vi "ClassPanel.vi"(8 "error in (no error)":errorcluster caption="entrée d'erreur (pas d'erreur)", 11 "ESP301.lvclass":refnum<class "ESP301.lvclass">) -> (0 "error out":errorcluster caption="sortie d'erreur", 3 "ESP301.lvclass Out":refnum<class "ESP301.lvclass">)   [LabVIEW 2019, in "ESP301.lvclass"]
uses:
  ESP301.lvclass
  C:/Programmes Labview/LabScanV1A/DevicesClass/BaseDevice/BaseDevice.lvclass
  ESP301.lvclass/ESP301.ctl
  BaseDevice/ClassQueueMess.ctl
  BaseDevice/Accessor/GetClassEvent.vi
panel:
  out "APDs":bool
  in  "Con/Disc.":bool
  in  "Enable":bool
  in  "Home":bool caption="MiseAJour"
  out "Moving":bool
  out "Axis Model":string
  out "Valid Ref":bool
  out "BKD Lim":bool
  out "FWD Lim":bool
  in  "Axis":u8(ring)=1 items=["1"=1, "2"=2, "3"=3]
  out "ActPos":dbl=60.0 caption="Actual Pos(mm)" min=0.1 step=0.1 format="%#.4f"
  in  "Target":dbl caption="Target(mm)" min=-25000.0 max=25000.0 step=0.0001 format="%#.4f"
  in  "Axis Name":string
  in  "MainProgQ":refnum<queue>
  in  "MainProgQEvent":refnum<user-event>
  in  "Acq":bool
  in  "Stop":bool
  in  "StopMotion":bool caption="MiseAJour"
  out "Init Program":bool
  # "this MUST labeled with class name"
  # "this MUST be present and labeled \"Stop\" and \"Acq\""
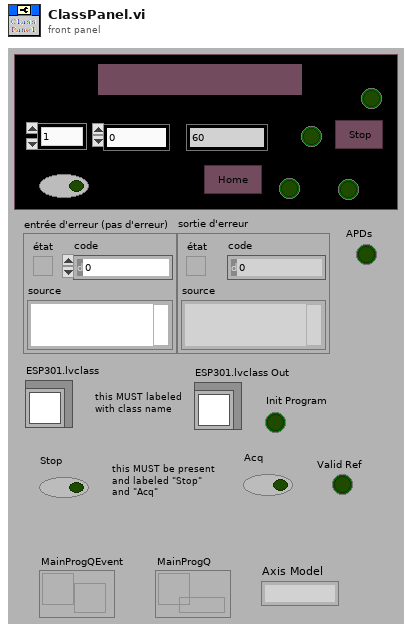
[diagram p1: front panel]
types:
  T1 = cluster{"ESP300mm":refnum<vi>, "ESP300ps":refnum<vi>, "MvgESP300":refnum<vi>}
  T2 = typedef "ClassQueueMess.ctl" = u16
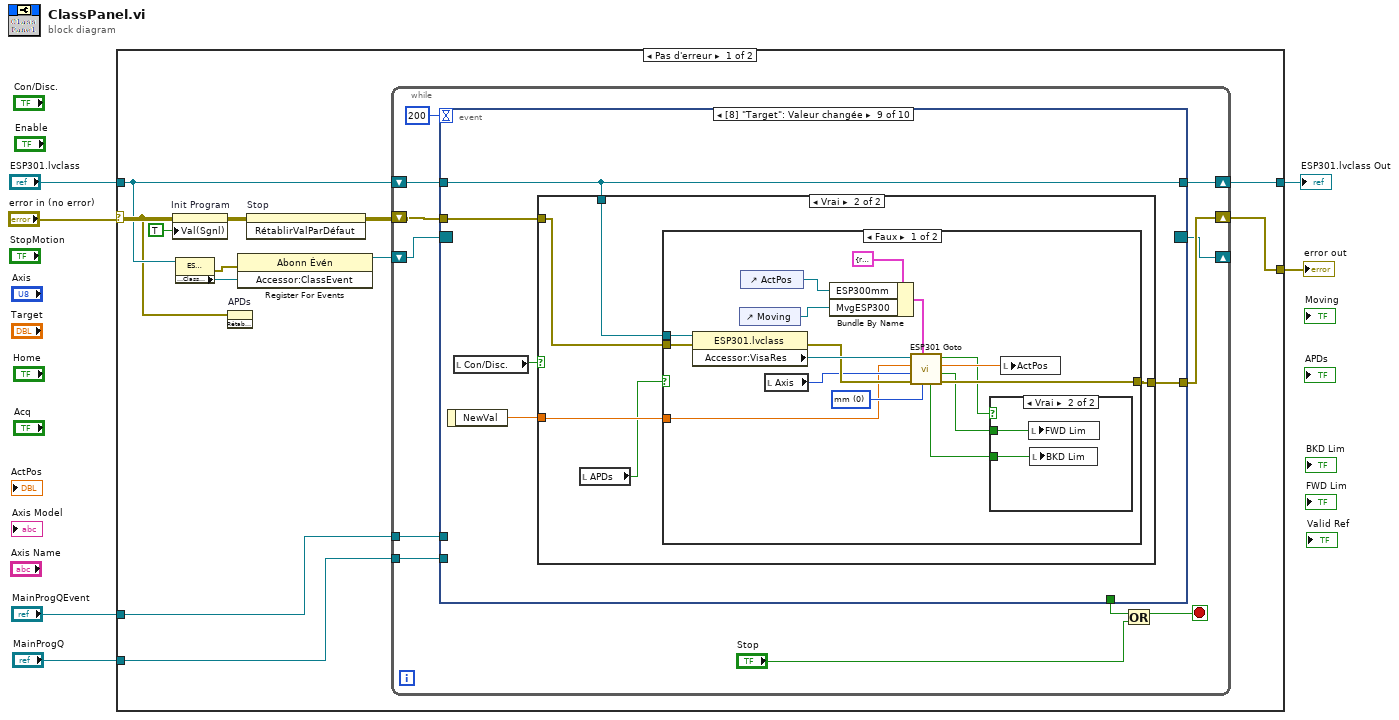
[diagram p0: block diagram]
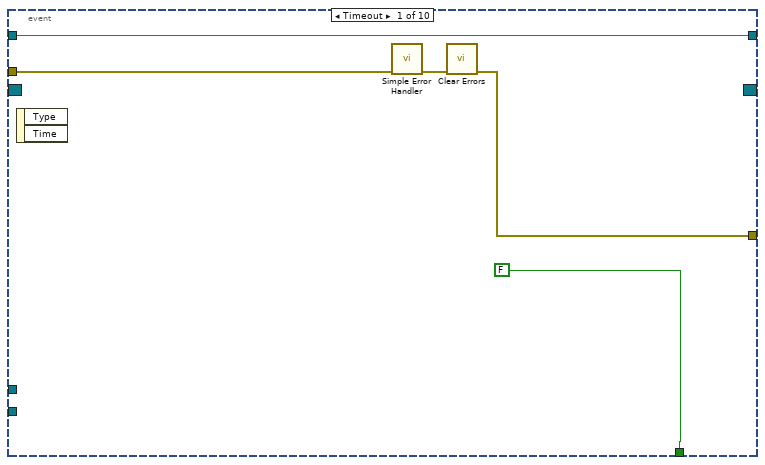
[diagram p2: hidden frame]
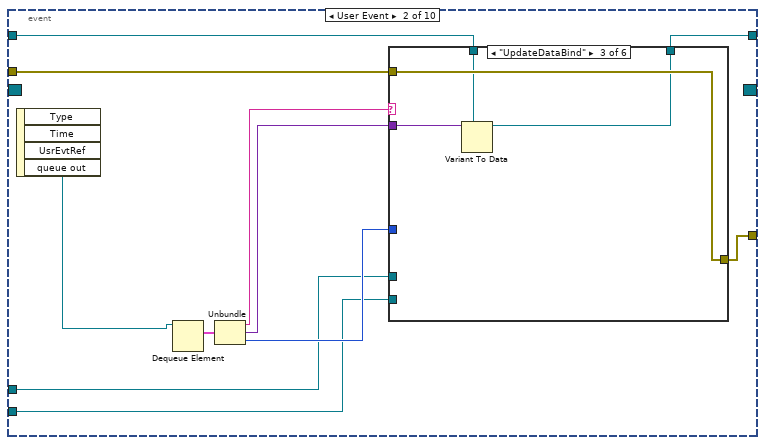
[diagram p3: hidden frame]
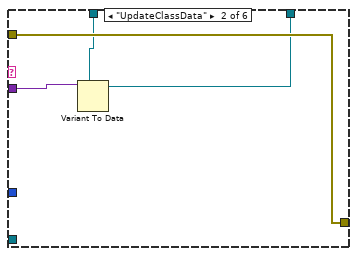
[diagram p5: hidden frame]
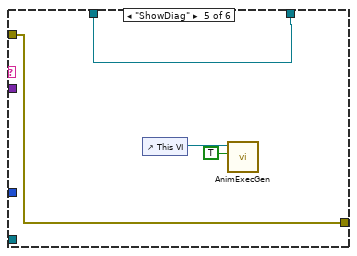
[diagram p7: hidden frame]
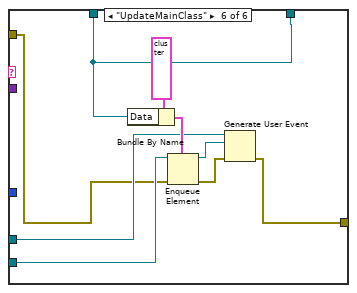
[diagram p8: hidden frame]
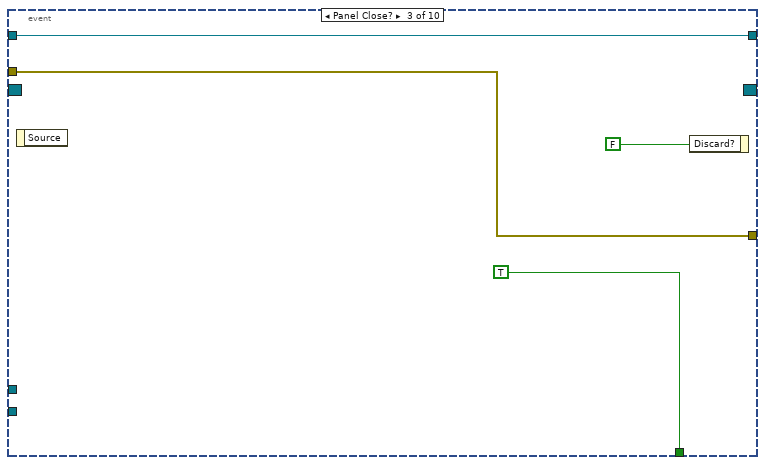
[diagram p9: hidden frame]
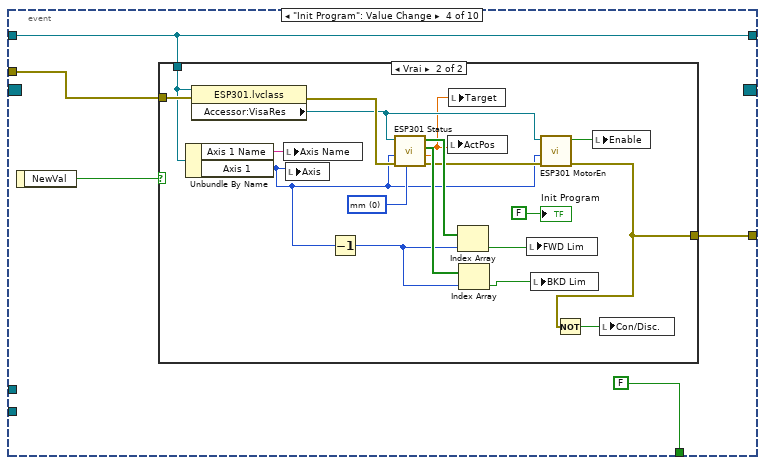
[diagram p10: hidden frame]
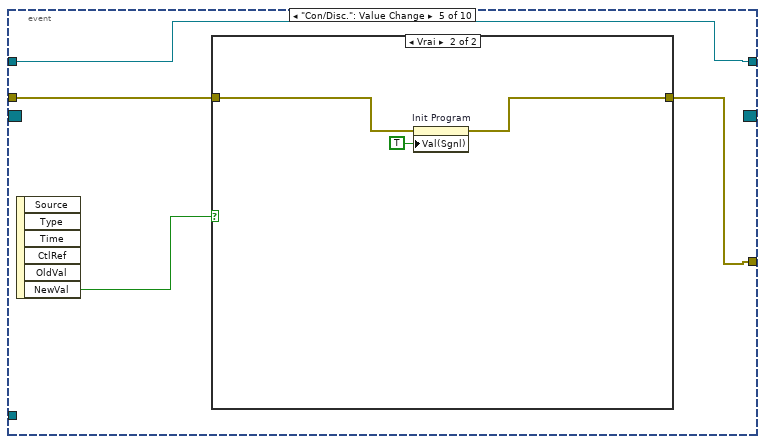
[diagram p12: hidden frame]
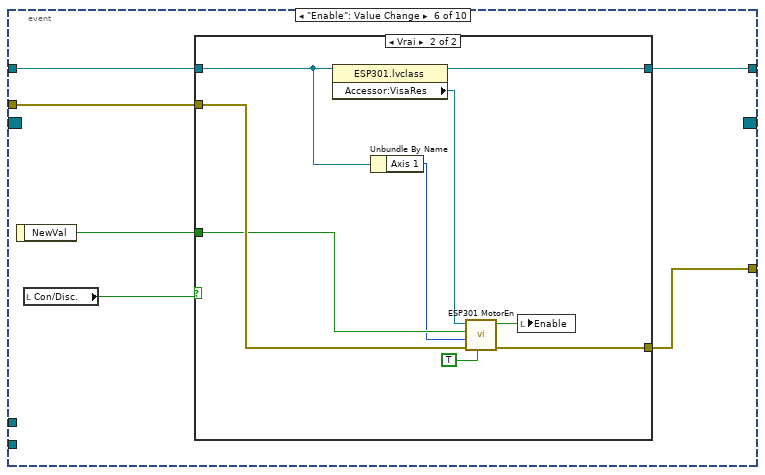
[diagram p14: hidden frame]
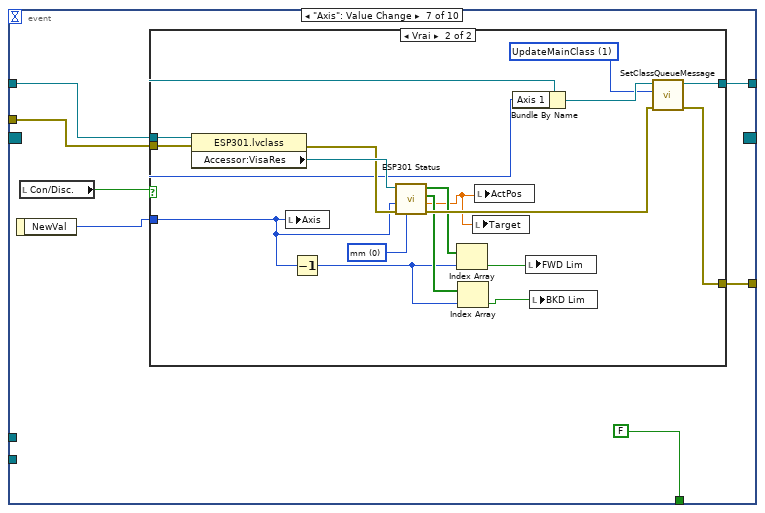
[diagram p16: hidden frame]
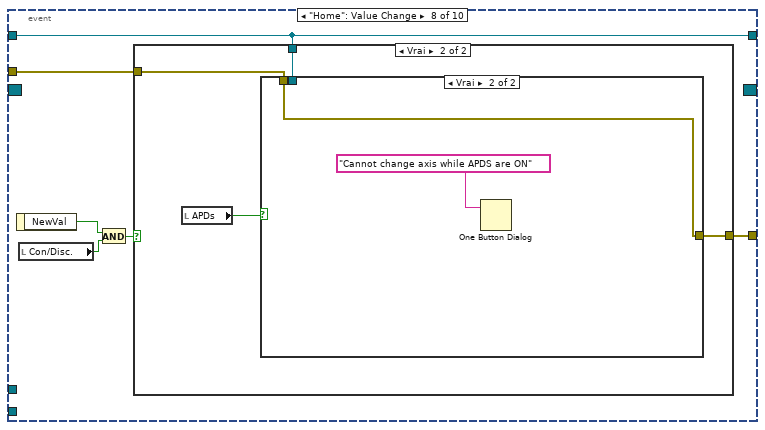
[diagram p18: hidden frame]
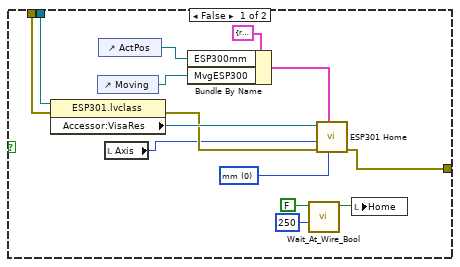
[diagram p20: hidden frame]
diagram:
  n1 = case shown="Pas d'erreur" "error in (no error)" {
    selector: "error in (no error)" -> [w7 w234]
    tunnel: [w18 w234] -> w5
    tunnel: "ESP301.lvclass" -> [w11 w233]
    tunnel: [w16 w233] -> w3
    tunnel: "MainProgQEvent" -> [w9 _]
    tunnel: "MainProgQ" -> [w8 _]
    frame No Error {
      n2 = property on="Init Program" class="Bool (strict)"(error in=w7, "Val(Sgnl)"=TRUE ("Valeur (Signalisation)")) -> (error out=w15:errorcluster)  [unwired: 1 in, 1 out]
      n3 = property class="ESP301.lvclass"(reference=w11) -> (error out=w13:errorcluster, "Accessor:ClassEvent"=w12:refnum<user-event>)  [unwired: 1 in, 1 out]
      n4 = invoke on="APDs" class="Bool (strict)" method="RétablirValParDéfaut"(error in=w7) -> ()  [unwired: 2 in, 3 out]
      n5 = register-events(error in=w13, w12) -> (reference out=w10:refnum<event-registration>)  [unwired: 1 in, 1 out]
      n6 = invoke on="Stop" class="Bool (strict)" method="RétablirValParDéfaut"(error in=w15) -> (error out=w14:errorcluster)  [unwired: 2 in, 2 out]
      n7 = while {
        shift-right: [w28] -> w18
        shift-left: w14 -> [w29]
        shift-right: [w26] -> w16
        shift-left: w11 -> [w27]
        shift-right: [w24] -> _
        shift-left: w10 -> [w25]
        tunnel: w9 -> [w23]
        tunnel: w8 -> [w22]
        stop <- w20 stop-if-true
        n8 = event shown="[8] \"Target\": Valeur changée" {
          selector: w25 -> [_ _ _ _ _ _ _ _ _ _]
          dyn-events: [_ _ _ _ _ _ _ _ _ _] -> w24
          timeout: 200 -> [_ _ _ _ _ _ _ _ _ _]
          tunnel: w29 -> [w33 w45 w73 w79 w102 w113 w131 w154 w181 w210]
          tunnel: [w31 w39 w73 w78 w103 w109 w127 w153 w180 w209] -> w28
          tunnel: w27 -> [w34 w46 w72 w76 w101 w110 w129 w155 w182 w211]
          tunnel: [FALSE _ TRUE FALSE _ _ FALSE _ _ _] -> w21
          tunnel: [w34 w38 w72 w76 w101 w111 w128 w155 w182 w212] -> w26
          tunnel: w23 -> [_ w37 _ _ _ _ _ _ _ _]
          tunnel: w22 -> [_ w36 _ _ _ _ _ _ _ _]
          event Timeout {
            n9 = event-data() -> ()  [unwired: 1 in, 2 out]
            n10 = call <vilib>:"Simple Error Handler.vi"("error in (no error)"=w33) -> ("error out"=w32:errorcluster)  [unwired: 4 in, 4 out]
            n11 = call <vilib>:"Clear Errors.vi"("error in (no error)"=w32) -> ("error out"=w31:errorcluster)  [unwired: 5 in, 1 out]
          }
          event User Event {
            n12 = event-data() -> ("queue out"=w43:refnum<queue>)  [unwired: 1 in, 3 out]
            n13 = Dequeue Element(queue=w43) -> (element=w44:cluster{"Message":string, "Data":variant, i32})  [unwired: 2 in, 3 out]
            n14 = Unbundle(w44) -> ("Message"=w42:string, "Data"=w41:variant, w40:i32)
            n15 = case shown="\"UpdateDataBind\"" w42 {
              tunnel: w45 -> [w48 w52 w56 w57 w61 w64]
              tunnel: w41 -> [_ w51 w55 _ _ _]
              tunnel: w46 -> [w47 w50 w54 w58 w62 w67]
              tunnel: [w47 w49 w53 w58 w62 w67] -> w38
              tunnel: [w48 w52 w56 w57 w61 w63] -> w39
              tunnel: w40 -> [_ _ _ _ _ _]
              tunnel: w37 -> [_ _ _ _ _ w66]
              tunnel: w36 -> [_ _ _ _ _ w65]
              frame Default {
              }
              frame "UpdateClassData" {
                n16 = Variant To Data(type=w50, Variant=w51) -> (data=w49:refnum<class "ESP301.lvclass">)  [unwired: 1 in, 1 out]
              }
              frame "UpdateDataBind" {
                n17 = Variant To Data(type=w54, Variant=w55) -> (data=w53:refnum<class "ESP301.lvclass">)  [unwired: 1 in, 1 out]
              }
              frame "MeasDone" {
              }
              frame "ShowDiag" {
                n18 = control-ref of="This VI"() -> (w60:refnum<vi>)
                n19 = call <userlib>:"AnimExecGen.vi"("Animer l'exécution ?"=TRUE, "ViRef"=w60) -> ()  [unwired: 9 in, 1 out]
              }
              frame "UpdateMainClass" {
                n20 = Bundle By Name(cluster=cluster{"Message":string, "Data":variant, i32} {"Message"="", "Data"=variant, 0} ("élément"), "Data"=w67) -> (w68:cluster{"Message":string, "Data":variant, i32})
                n21 = Enqueue Element(queue=w65, element=w68, error in (no error)=w64) -> (queue out=w71:refnum<queue>, error out=w70:errorcluster)  [unwired: 1 in, 1 out]
                n22 = Generate User Event(user event=w66, event data cluster=w71, error in=w70) -> (error out=w63:errorcluster)  [unwired: 1 in, 1 out]
              }
            }
          }
          event Panel Close? {
            n23 = event-data() -> ()  [unwired: 1 in, 1 out]
            n24 = event-data("Discard?"=FALSE ("Rejeter ?")) -> ()  [unwired: 1 in, 1 out]
          }
          event "Init Program": Value Change {
            n25 = event-data() -> ("NewVal"=w80:bool)  [unwired: 1 in]
            n26 = case shown="Vrai" w80 {
              tunnel: w79 -> [w81 w98]
              tunnel: [w81 w83] -> w78
              tunnel: w76 -> [_ w97]
              frame False {
              }
              frame True {
                w94 = i8 0 items=["mm", "ps"] ("Input Units")
                n27 = Unbundle By Name(w97) -> ("Axis 1 Name"=w96:string, "Axis 1"=w87:u8)
                n28 = property class="ESP301.lvclass"(reference=w97, error in=w98) -> (error out=w95:errorcluster, "Accessor:VisaRes"=w88:refnum<visa-resource-name>)  [unwired: 1 out]
                n29 = local write "Axis Name"(w96) -> ()
                n30 = local write "Axis"(w87) -> ()
                n31 = Decrement(x=w87) -> (x-1=w85:u8)
                n32 = call <userlib>:"ESP301 Status.vi"("Input Units"=w94, "error in"=w95, "Axis"=w87, "VISA Rsrc"=w88) -> ("error out"=w89:errorcluster, "Position"=w84:dbl, "Low Limit"=w90:bool[], "High Limit"=w91:bool[])  [unwired: 4 in]
                n33 = local write "ActPos"(w84) -> ()
                n34 = local write "Target"(w84) -> ()
                n35 = Index Array(array=w91, index=w85) -> (element=w92:bool)
                n36 = Index Array(array=w90, index=w85) -> (element=w93:bool)
                n37 = local write "FWD Lim"(w92) -> ()
                n38 = local write "BKD Lim"(w93) -> ()
                n39 = call <userlib>:"ESP301 MotorEn.vi"("error in"=w89, "Axis"=w87, "VISA Rsrc"=w88) -> ("error out"=w83:errorcluster, "MotorEnOut"=w86:bool)  [unwired: 7 in]
                n40 = Not(x=w83) -> (.not. x?=w82:bool)
                n41 = local write "Enable"(w86) -> ()
                n42 = local write "Con/Disc."(w82) -> ()
                "Init Program" <- FALSE
              }
            }
          }
          event "Con/Disc.": Value Change {
            n43 = event-data() -> ("NewVal"=w100:bool)  [unwired: 1 in, 5 out]
            n44 = case shown="Vrai" w100 {
              tunnel: [w104 w105] -> w103
              tunnel: w102 -> [w104 w106]
              frame False {
              }
              frame True {
                n45 = property on="Init Program" class="Bool (strict)"(error in=w106, "Val(Sgnl)"=TRUE ("Valeur (Signalisation)")) -> (error out=w105:errorcluster)  [unwired: 1 in, 1 out]
              }
            }
          }
          event "Enable": Value Change {
            n46 = event-data() -> ("NewVal"=w112:bool)  [unwired: 1 in]
            n47 = local read "Con/Disc."() -> (w108:bool)
            n48 = case shown="Vrai" w108 {
              tunnel: w113 -> [w114 w123]
              tunnel: w112 -> [_ w120]
              tunnel: [w115 w119] -> w111
              tunnel: w110 -> [w115 w118]
              tunnel: [w114 w116] -> w109
              frame False {
              }
              frame True {
                n49 = property class="ESP301.lvclass"(reference=w118) -> (reference out=w119:refnum<class "ESP301.lvclass">, "Accessor:VisaRes"=w122:refnum<visa-resource-name>)  [unwired: 1 in, 1 out]
                n50 = Unbundle By Name(w118) -> ("Axis 1"=w117:u8)
                n51 = call <userlib>:"ESP301 MotorEn.vi"("Set"=TRUE, "error in"=w123, "Axis"=w117, "MotorEn"=w120, "VISA Rsrc"=w122) -> ("error out"=w116:errorcluster, "MotorEnOut"=w124:bool)  [unwired: 5 in]
                n52 = local write "Enable"(w124) -> ()
              }
            }
          }
          event "Axis": Value Change {
            n53 = event-data() -> ("NewVal"=w126:u8)  [unwired: 1 in]
            n54 = local read "Con/Disc."() -> (w125:bool)
            n55 = case shown="Vrai" w125 {
              tunnel: w131 -> [w132 w150]
              tunnel: w129 -> [w133 w149]
              tunnel: [w133 w147] -> w128
              tunnel: [w132 w146] -> w127
              tunnel: w126 -> [_ w136]
              frame False {
              }
              frame True {
                w145 = T2 1 items=["UpdateClassData", "UpdateMainClass", "UpdateDataBind", "ReInitDevice", "Custom", "ClosePan"] ("Menu déroulant")
                w141 = i8 0 items=["mm", "ps"] ("Input Units")
                n56 = property class="ESP301.lvclass"(reference=w149, error in=w150) -> (error out=w143:errorcluster, "Accessor:VisaRes"=w144:refnum<visa-resource-name>)  [unwired: 1 out]
                n57 = local write "Axis"(w136) -> ()
                n58 = Decrement(x=w136) -> (x-1=w135:u8)
                n59 = call <userlib>:"ESP301 Status.vi"("Input Units"=w141, "error in"=w143, "Axis"=w136, "VISA Rsrc"=w144) -> ("error out"=w142:errorcluster, "Position"=w134:dbl, "Low Limit"=w137:bool[], "High Limit"=w140:bool[])  [unwired: 4 in]
                n60 = Index Array(array=w140, index=w135) -> (element=w138:bool)
                n61 = Index Array(array=w137, index=w135) -> (element=w139:bool)
                n62 = local write "Target"(w134) -> ()
                n63 = local write "ActPos"(w134) -> ()
                n64 = Bundle By Name(cluster=w149, "Axis 1"=w136) -> (w148:refnum<class "ESP301.lvclass">)
                n65 = local write "FWD Lim"(w138) -> ()
                n66 = local write "BKD Lim"(w139) -> ()
                n67 = call-dynamic "SetClassQueueMessage.vi"("ErrorIn(No Error)"=w142, "Menu déroulant"=w145, "DefaultDev.lvclass"=w148) -> ("sortie d'erreur"=w146:errorcluster, "DefaultDev.lvclass Out"=w147:refnum<class "ESP301.lvclass">)  [unwired: 7 in]
              }
            }
          }
          event "Home": Value Change {
            n68 = event-data() -> ("NewVal"=w156:bool)  [unwired: 1 in]
            n69 = local read "Con/Disc."() -> (w151:bool)
            n70 = And(x=w156, y=w151) -> (x .and. y?=w152:bool)
            n71 = case shown="Vrai" w152 {
              tunnel: w155 -> [_ w159]
              tunnel: w154 -> [w157 w161]
              tunnel: [w157 w160] -> w153
              frame False {
              }
              frame True {
                n72 = local read "APDs"() -> (w158:bool)
                n73 = case shown="Vrai" w158 {
                  tunnel: w161 -> [w168 w176]
                  tunnel: [w166 w176] -> w160
                  tunnel: w159 -> [w162 _]
                  frame False {
                    w172 = i8 0 items=["mm", "ps"] ("Input Units")
                    n74 = property class="ESP301.lvclass"(reference=w162, error in=w168) -> (error out=w174:errorcluster, "Accessor:VisaRes"=w175:refnum<visa-resource-name>)  [unwired: 1 out]
                    n75 = control-ref of="Moving"() -> (w167:refnum<vi>)
                    n76 = control-ref of="ActPos"() -> (w170:refnum<vi>)
                    n77 = local read "Axis"() -> (w173:u8)
                    n78 = Bundle By Name(cluster=T1 {"ESP300mm"=refnum, "ESP300ps"=refnum, "MvgESP300"=refnum} ("ESP301Ref"), "ESP300mm"=w170, "MvgESP300"=w167) -> (w169:T1)
                    n79 = call <userlib>:"Wait_At_Wire_Bool.vi"("Wait (ms)"=u32 250, "error in (no error)"=FALSE) -> ("error out"=w165:bool)  [unwired: 7 in, 2 out]
                    n80 = call <userlib>:"ESP301 Home.vi"("Input Units"=w172, "ESP301Ref"=w169, "error in"=w174, "Axis"=w173, "VISA Rsrc"=w175) -> ("error out"=w166:errorcluster)  [unwired: 6 in]
                    n81 = local write "Home"(w165) -> ()
                  }
                  frame True {
                    n82 = One Button Dialog(message="Cannot change axis while APDS are ON") -> ()  [unwired: 1 in, 1 out]
                  }
                }
              }
            }
          }
          event "Target": Value Change {
            n83 = event-data() -> ("NewVal"=w179:dbl)  [unwired: 1 in]
            n84 = local read "Con/Disc."() -> (w178:bool)
            n85 = case shown="Vrai" w178 {
              tunnel: w182 -> [_ w188]
              tunnel: w181 -> [w183 w185]
              tunnel: [w183 w187] -> w180
              tunnel: w179 -> [_ w186]
              frame False {
              }
              frame True {
                n86 = local read "APDs"() -> (w184:bool)
                n87 = case shown="Faux" w184 {
                  tunnel: w188 -> [w204 _]
                  tunnel: [w197 w208] -> w187
                  tunnel: w186 -> [w196 _]
                  tunnel: w185 -> [w189 w208]
                  frame False {
                    w198 = i8 0 items=["mm", "ps"] ("Input Units")
                    n88 = property class="ESP301.lvclass"(reference=w204, error in=w189) -> (error out=w200:errorcluster, "Accessor:VisaRes"=w201:refnum<visa-resource-name>)  [unwired: 1 out]
                    n89 = control-ref of="Moving"() -> (w202:refnum<vi>)
                    n90 = control-ref of="ActPos"() -> (w203:refnum<vi>)
                    n91 = local read "Axis"() -> (w199:u8)
                    n92 = Bundle By Name(cluster=T1 {"ESP300mm"=refnum, "ESP300ps"=refnum, "MvgESP300"=refnum} ("ESP301Ref"), "ESP300mm"=w203, "MvgESP300"=w202) -> (w191:T1)
                    n93 = call <userlib>:"ESP301 Goto.vi"("Input Units"=w198, "ESP301Ref"=w191, "error in"=w200, "Axis"=w199, "Position"=w196, "VISA Rsrc"=w201) -> ("error out"=w197:errorcluster, "HighLim"=w193:bool, "Pos Out"=w195:dbl, "Warning"=w192:bool, "LowLim"=w194:bool)  [unwired: 1 in]
                    n94 = case shown="Vrai" w192 {
                      tunnel: w194 -> [_ w206]
                      tunnel: w193 -> [_ w205]
                      frame False {
                      }
                      frame True {
                        n95 = local write "FWD Lim"(w205) -> ()
                        n96 = local write "BKD Lim"(w206) -> ()
                      }
                    }
                    n97 = local write "ActPos"(w195) -> ()
                  }
                  frame True {
                    n98 = One Button Dialog(message="Cannot change axis while APDS are ON") -> ()  [unwired: 1 in, 1 out]
                  }
                }
              }
            }
          }
          event "Axis Name": Shortcut Menu Selection (User) {
            n99 = event-data() -> ("ItemTag"=w213:string)  [unwired: 1 in]
            n100 = case shown="\"ChangeName\"" w213 {
              tunnel: [w215 w220] -> w212
              tunnel: w211 -> [w215 w221]
              tunnel: w210 -> [w214 w222]
              tunnel: [w214 w217] -> w209
              frame Default {
              }
              frame "ChangeName" {
                n101 = call "SaveAxisName"("Enable"=TRUE, "error in (no error)"=w222) -> ("Name"=w216:string, "Save"=w219:bool, "error out"=w218:errorcluster)  [unwired: 15 in]
                n102 = case shown="Vrai" w219 {
                  tunnel: w221 -> [w225 w232]
                  tunnel: [w225 w230] -> w220
                  tunnel: w218 -> [w224 w229]
                  tunnel: [w224 w228] -> w217
                  tunnel: w216 -> [_ w227]
                  frame False {
                  }
                  frame True {
                    w226 = T2 1 items=["UpdateClassData", "UpdateMainClass", "UpdateDataBind", "ReInitDevice", "Custom", "ClosePan"] ("Menu déroulant")
                    n103 = Bundle By Name(cluster=w232, "Axis 1 Name"=w227) -> (w231:refnum<class "ESP301.lvclass">)
                    n104 = local write "Axis Name"(w227) -> ()
                    n105 = call-dynamic "SetClassQueueMessage.vi"("ErrorIn(No Error)"=w229, "Menu déroulant"=w226, "DefaultDev.lvclass"=w231) -> ("sortie d'erreur"=w228:errorcluster, "DefaultDev.lvclass Out"=w230:refnum<class "ESP301.lvclass">)  [unwired: 7 in]
                  }
                }
              }
            }
          }
        }
        n106 = Or(x=w21, y="Stop") -> (x .or. y?=w20:bool)
      }
    }
    frame Error {
    }
  }
  "error out" <- w5
  "ESP301.lvclass Out" <- w3
